vi "Nicolet 12 ICAI_gatefix3.vi"(3 "?":u16(ring)=10 items=["16", "32", "64", "128", "256", "512", "1024", "2048", "4096", "8192", "16384", "32768", "65536", "131072", "262144", "524288 (one channel)", ""], 5 "Sample Duration (sec)":u32(knob)=24 scale=1.0..33.0) -> (0 "Waveform Graph":waveform(dbl)[](graph)=[{"t0"=timestamp(0 s since 1904-01-01), "dt"=0.0001220703125, "Y"=array[40960 elements]}, {"t0"=timestamp(0 s since 1904-01-01), "dt"=0.0001220703125, "Y"=array[40960 elements]}], 2 "data":dbl[][](array[numeric]) format="%0.2f", 8 "points":i32=40960)   [LabVIEW 2010]
doc: "I. Description:\nThis example demonstrates how to acquire a finite amount of data (Waveform) using the DAQ device's internal clock, started by an analog edge condition.\n\nII. Instructions for Running:\n1. Select the physical channel to correspond to where your signal is input on the DAQ device.\n2. Enter the minimum and maximum voltage range.\nNote: For better accuracy try to match the input range to the expected voltage level of the measured signal.\n3. Set the number of samples to acquire per channel.\n4. Set the rate of the acquisition\nNote: The rate should be AT LEAST twice as fast as the maximum frequency component of the signal being acquired.\n5. Set the source of the start trigger. By default this is PFI0\n6. Set the slope and level of desired analog edge condition.\n\nIII. Block Diagram Steps:\n1. Create an empty task.\n2. Create an analog input voltage channel.\n3. Set the rate for the sample clock. Additionally, define the sample mode to be finite.\n4. Define the parameters for an Analog Slope Start Trigger.\n5. Call the Start VI to start the acquisition.\n6. Read all of the data.\n7. Stop the Analog Input Task.\n8. Call the Clear Task VI to clear the Task.\n9. Use the popup dialog box to display an error if any\nIV. I/O Connections Overview:\nMake sure your signal input terminal matches the Physical Channel I/O Control. In this case wire your signal to the ai0 pin on your DAQ Device."
uses:
  programs/Detection/200262.llb/Trigger Select.ctl
  <vilib>/Utility/error.llb/DialogType.ctl
  <vilib>/DAQmx/write.llb/DAQmx Write (Analog DBL 1Chan 1Samp).vi
  <vilib>/DAQmx/read.llb/DAQmx Read (Analog 2D DBL NChan NSamp).vi
  <vilib>/DAQmx/create/channels.llb/DAQmx Create Channel (AO-Voltage-Basic).vi
  <vilib>/daqmx/miscellaneous.llb/DAQmx Fill In Error Info.vi
  <vilib>/DAQmx/create/channels.llb/DAQmx Create Channel (AI-Voltage-Basic).vi
  <vilib>/DAQmx/configure/timing.llb/DAQmx Timing (Sample Clock).vi
  <vilib>/DAQmx/configure/trigger.llb/DAQmx Start Trigger (Analog Edge).vi
  <vilib>/DAQmx/configure/trigger.llb/DAQmx Reference Trigger (Digital Edge).vi
  <vilib>/measure/maspectr.llb/FFT Power Spectral Density for 1 Chan.vi
  <vilib>/measure/NI_MAPro.lvlib
  Program Files/National Instruments/LabVIEW 2010/resource/objmgr/daqmx.rc
panel:
  out "size(s)":i32[](array[numeric])
  in  "CAI/ICAI":bool=TRUE
  in  "?":path=path "C:/Users/Cardenas/Desktop/7_01/7_01_380fringe371mvmid_lockedat330.txt"
  in  "Path":path=path "C:/Users/Cardenas/Desktop/7_03/a6_200ms_span.txt"
  out "Time":dbl=5.5
  out "points pretriger":dbl=4096.0
  in  "Iterations to Average":i32=8
  in  "Sample Rate Hz":bool
  out "Cursor Time Selected":dbl=0.22413589186805782
  out "Cursor Peak to Peak Voltage":dbl=0.01024955436720143
  in  "Save Average To File":bool
  out "Pretrigger Samples":dbl=4096.0
  out "Seconds Per Division":dbl=0.1
  out "Posttrigger Samples Captured":dbl=40960.0
  in  "Voltage Offset":dbl(knob) scale=-2.0..2.0
  in  "Average / Live Display":bool
  in  "Seconds  Per Division":u32(knob) min=1 max=1 step=1 scale=0.0..15.0
  out "Samples Averaged":i32=3
  in  "?":bool=TRUE
  in  "Volts Per Division":dbl(knob)=0.5 scale=0.005..5.0
  in  "Pretrigger Duration (%)":dbl(knob)=0.1 min=0.0 max=2.0 step=1.0 scale=0.05..0.95
  in  "Analog Source":string="APFI0"
  in  "Digital External TTL Source":tag="/Dev1/PFI13"
  in  "Trigger Type":T1=enum."Digital Edge"
  in  "Analog Edge Level":dbl=-0.1 format="%0.2f"
  in  "Edge":i32(ring)=10280 items=["Rising"=10280, "Falling"=10171]
  in  "Physical Channel":tag="Dev1/ai22, Dev1/ai23" caption="Physical Channels"
  out "Sampling Iterations":i32=2
  in  "Maximum  Voltage":dbl=10.0
  in  "Minimum Voltage":dbl=-10.0
  out "Sampling Rate":i32=8192 caption="Sample Rate (Hz)"
  in  "stop":bool
  # "Channel\nConfiguration"
  # "Triggering Parameters"
  # "Voltage Parameters"
  # "TTL Trigger Options"
  # "Timing Parameters"
  # "External  Trigger Options"
  # "Storage Options"
  # "Nicolet 8.vi*If X scale markers are not drawn:\nRight click the waveform diagram -> select X axis -> marker spacing -> set to arbitrary AFTER\nsetting the correct seconds per division"
  # "CAI / ICAI"
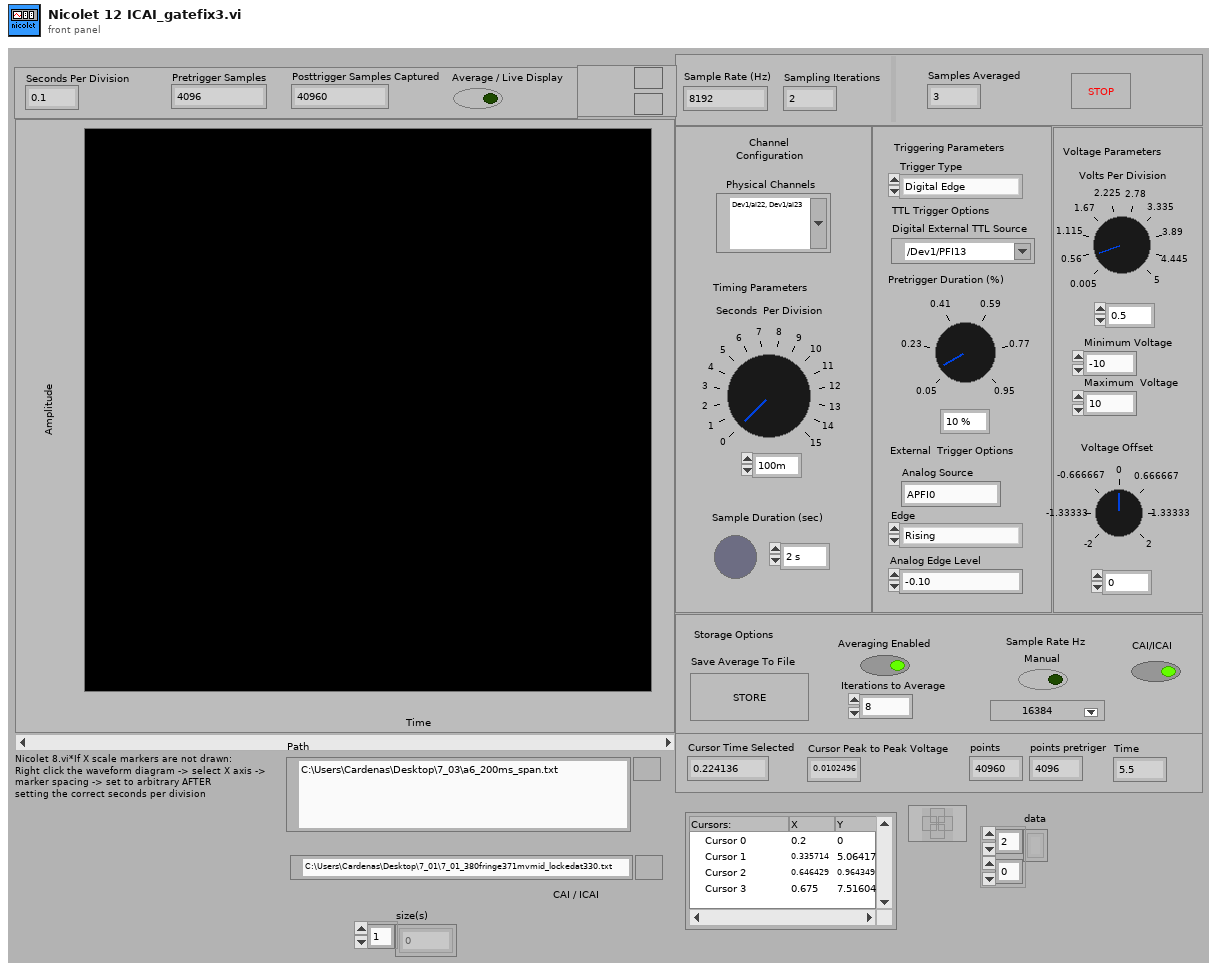
[diagram p1: front panel]
types:
  T1 = typedef "Trigger Select.ctl" = enum16{"None", "Analog Edge", "Digital Edge"}
  T2 = typedef "DialogType.ctl" = u16
  T3 = typedef "LVCursorListTypeDef.ctl" = cluster{"Name":string, "Color":u32, "Style":u8, "Point Style":u8, "Name Visible":bool, "Allow Drag":bool, "Cursor Mode":u32, "Plot":i32, "Index":i32, "Position":cluster{"X":dbl, "Y":dbl}, "X Scale":u32, "Y Scale":u32, "Watch Plots":i32[], "Watch All Plots":bool, "Plot Area":i32, "Label Offset":cluster{"X":dbl, "Y":dbl}}[]
  T4 = cluster{"Name":string, "Color":u32, "Style":u8, "Point Style":u8, "Name Visible":bool, "Allow Drag":bool, "Cursor Mode":u32, "Plot":i32, "Index":i32, "Position":cluster{"X":dbl, "Y":dbl}, "X Scale":u32, "Y Scale":u32, "Watch Plots":i32[], "Watch All Plots":bool, "Plot Area":i32, "Label Offset":cluster{"X":dbl, "Y":dbl}}
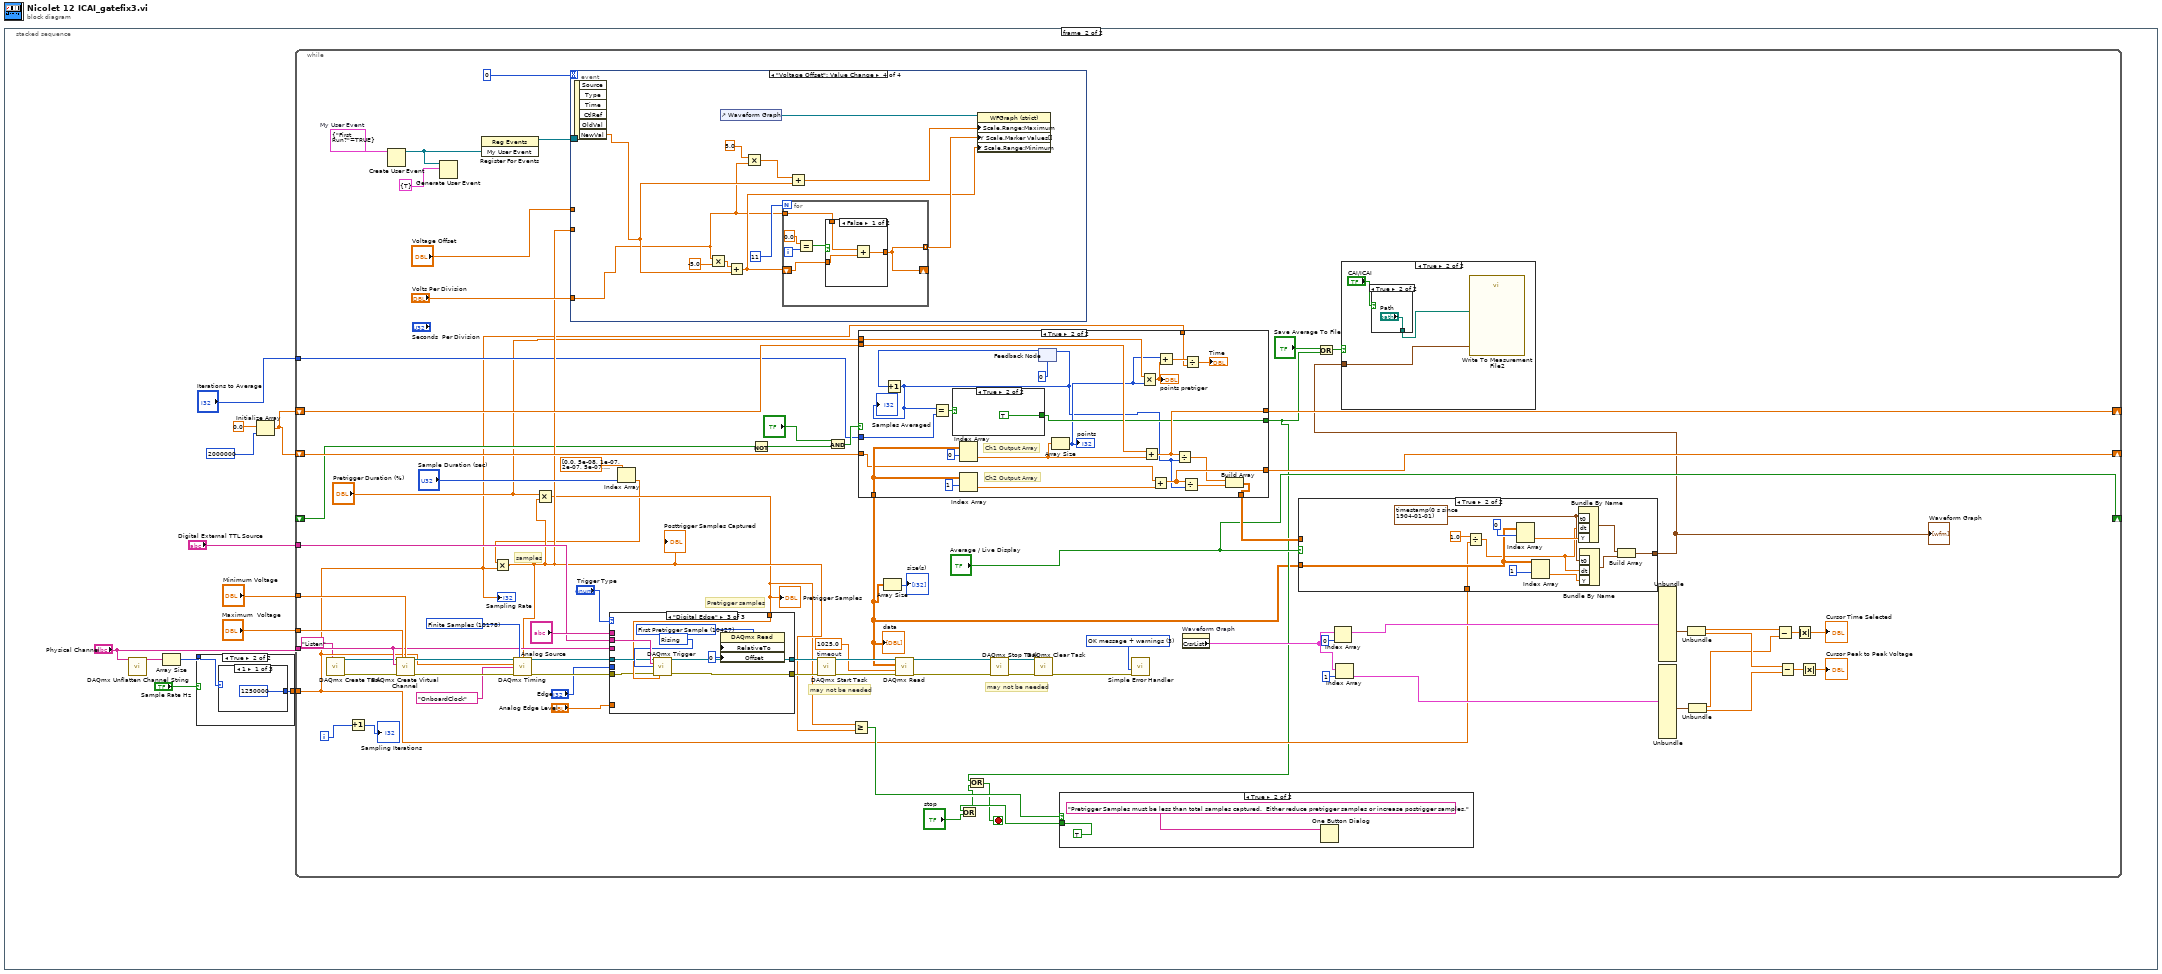
[diagram p0: block diagram]
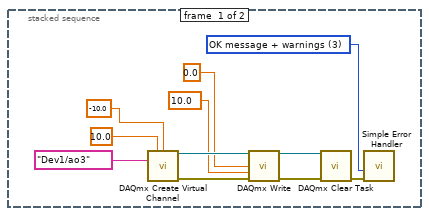
[diagram p2: hidden frame]
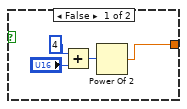
[diagram p3: hidden frame]
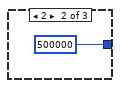
[diagram p4: hidden frame]
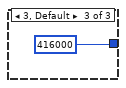
[diagram p5: hidden frame]
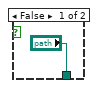
[diagram p7: hidden frame]
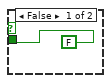
[diagram p8: hidden frame]
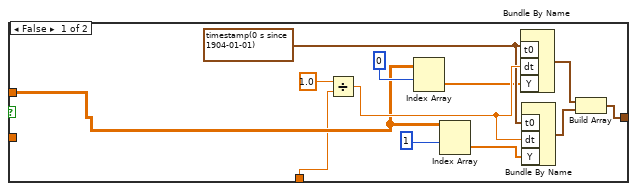
[diagram p9: hidden frame]
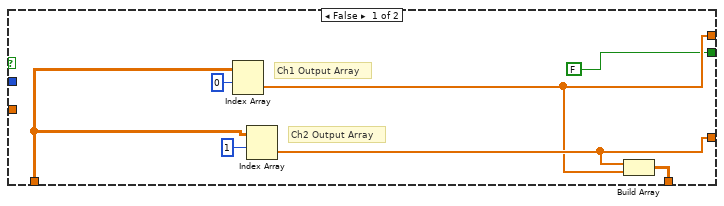
[diagram p10: hidden frame]
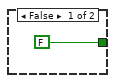
[diagram p11: hidden frame]
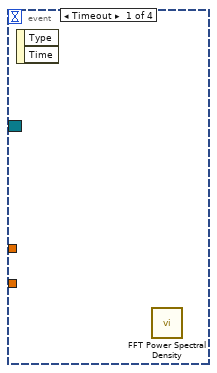
[diagram p12: hidden frame]
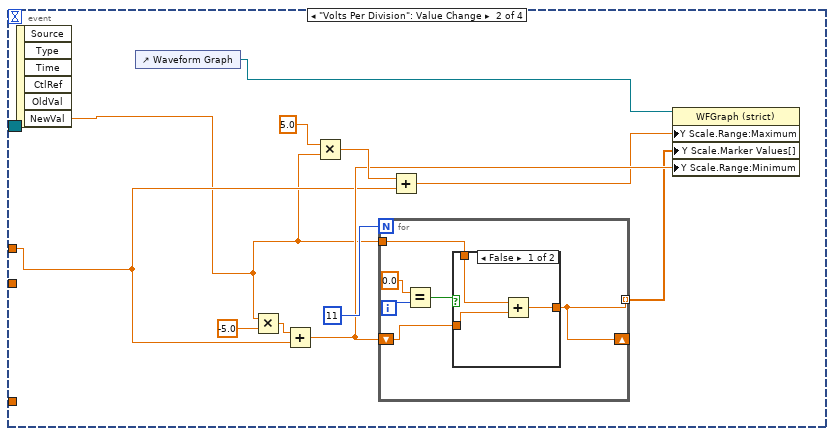
[diagram p13: hidden frame]
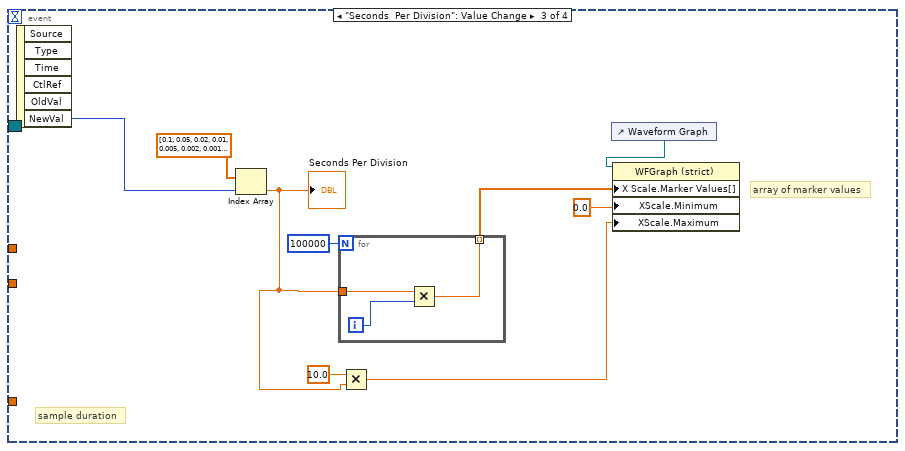
[diagram p15: hidden frame]
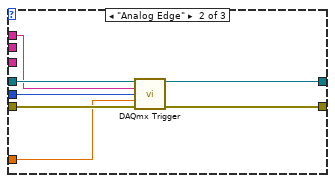
[diagram p18: hidden frame]
diagram:
  n1 = stacked-sequence {
    frame #0 {
      w4 = T2 3 items=["no dialog", "OK message", "continue or stop message", "OK message + warnings", "continue/stop + warnings"] ("type of dialog (OK msg:1)")
      n2 = call-poly <vilib>:"DAQmx Create Virtual Channel.vi"("maximum value"=10.0 ("Maximum Value"), "minimum value"=-10.0 ("Minimum Value"), "physical channels"=tag "Dev1/ao3" ("Physical Channel")) -> ("task out"=w7:refnum<k21>, "error out"=w8:errorcluster)  [unwired: 6 in, 5 out]
      n3 = call-poly <vilib>:"DAQmx Write.vi"("task/channels in"=w7, "data"=0.0 ("Voltage Output"), "timeout"=10.0, "error in"=w8) -> ("task out"=w2:refnum<k21>, "error out"=w3:errorcluster)  [unwired: 1 in, 9 out]
      n4 = call <vilib>:"DAQmx Clear Task.vi"("task in"=w2, "error in"=w3) -> ("error out"=w1:errorcluster)  [unwired: 13 out]
      n5 = call <vilib>:"Simple Error Handler.vi"("type of dialog (OK msg:1)"=w4, "error in (no error)"=w1) -> ()  [unwired: 8 out]
    }
    frame #1 {
      n6 = call <vilib>:"DAQmx Unflatten Channel String.vi"("names in"="Physical Channel") -> ("names out"=w19:string[])  [unwired: 1 in, 13 out]
      n7 = Array Size(array=w19) -> (size(s)=w17:i32)
      n8 = case shown="True" "Sample Rate Hz" {
        tunnel: [w25 w29] -> w18
        tunnel: w17 -> [_ w28]
        frame False {
          n9 = Add(x=4, y="?") -> (x+y=w26:i32)
          n10 = Power Of 2(x=w26) -> (2^x=w25:dbl)
        }
        frame True {
          n11 = case shown="1" w28 {
            tunnel: [1250000 500000 416000] -> w29
            frame 1 {
            }
            frame 2 {
            }
            frame 3, Default {
            }
          }
        }
      }
      n12 = Initialize Array(0.0, 2000000) -> (w12:dbl[])
      n13 = while {
        tunnel: "Minimum Voltage" -> [w94]
        tunnel: "Maximum  Voltage" -> [w93]
        tunnel: "Physical Channel" -> [w92]
        tunnel: "Digital External TTL Source" -> [w90]
        shift-right: [w84] -> _
        shift-left: w12 -> [w83]
        shift-right: [w79] -> _
        shift-left: w12 -> [w78]
        tunnel: w18 -> [w41]
        shift-right: ["Average / Live Display"] -> _
        shift-left: _ -> [w51]
        tunnel: "Iterations to Average" -> [w43]
        i -> [w37]
        stop <- w40 stop-if-true
        w89 = cluster{"First Run?":bool} {"First Run?"=TRUE}  # My User Event
        w109 = T2 3 items=["no dialog", "OK message", "continue or stop message", "OK message + warnings", "continue/stop + warnings"] ("type of dialog (OK msg:1)")
        w106 = 1025.0  # timeout
        w104 = 10178 items=["Finite Samples"=10178, "Continuous Samples"=10123] ("sample mode")
        # "samples"
        # "may not be needed"
        # "may not be needed"
        # "Pretrigger samples"
        n14 = call <vilib>:"DAQmx Create Task.vi"("new task name"="Listen") -> ("task out"=w82:refnum<k21>, "error out"=w81:errorcluster)  [unwired: 4 in, 9 out]
        n15 = Increment(x=w37) -> (x+1=→"Sampling Iterations":i32)
        n16 = Create User Event(user event datatype=w89) -> (user event=w87:refnum<user-event>)  [unwired: 1 in, 1 out]
        n17 = call-poly <vilib>:"DAQmx Create Virtual Channel.vi"("task in"=w82, "maximum value"=w93, "minimum value"=w94, "physical channels"=w92, "error in"=w81) -> ("task out"=w105:refnum<k21>, "error out"=w113:errorcluster)  [unwired: 4 in, 5 out]
        n18 = Generate User Event(user event=w87, event data cluster=cluster{"First Run?":bool} {"First Run?"=TRUE} ("event data")) -> ()  [unwired: 1 in, 2 out]
        n19 = register-events(w87) -> (reference out=w85:refnum<event-registration>)  [unwired: 2 in, 1 out]
        n20 = Index Array(array=dbl[] [0.0, 5e-08, 1e-07, 2e-07, 5e-07, 1e-06, 2e-06, 5e-06, 1e-05, 2e-05, 5e-05, 0.0001, 0.0002, 0.0005, 0.001, 0.002, 0.005, 0.01, 0.02, 0.05, 0.1, 0.2, 0.5, 1.0, 2.0, 5.0, 10.0, 16.5, 32.5, 65.0, 129.0, 257.0, 513.0, 1025.0], index="Sample Duration (sec)") -> (element=w48:dbl)
        n21 = Multiply(x=w48, y=w41) -> (x*y=w70:dbl)
        "Posttrigger Samples Captured" <- w70
        n22 = call-poly <vilib>:"DAQmx Timing.vi"("task/channels in"=w105, "sample mode"=w104, "samples per channel"=w70, "rate"=w41, "source"=tag "OnboardClock", "error in"=w113) -> ("task out"=w99:refnum<k21>, "error out"=w97:errorcluster)  [unwired: 1 in, 7 out]
        n23 = Multiply(x="Pretrigger Duration (%)", y=w70) -> (x*y=w69:dbl)
        "Pretrigger Samples" <- w69
        n24 = event shown="[3] \"Voltage Offset\": Value Change" {
          selector: w85 -> [_ _ _ _]
          dyn-events: _ -> [_ _ _ _]
          timeout: 0 -> [_ _ _ _]
          tunnel: w70 -> [_ _ _ _]
          tunnel: "Voltage Offset" -> [_ w181 _ _]
          tunnel: "Volts Per Division" -> [_ _ _ w213]
          event Timeout {
            n25 = event-data() -> ()  [unwired: 3 out]
            n26 = call-poly <vilib>:"FFT Power Spectral Density.vi"() -> ()  [unwired: 6 in, 6 out]
          }
          event "Volts Per Division": Value Change {
            n27 = event-data() -> ("NewVal"=w180:dbl)  [unwired: 6 out]
            n28 = control-ref of="Waveform Graph"() -> (w179:refnum<vi>)
            n29 = Multiply(x=w180, y=-5.0) -> (x*y=w186:dbl)
            n30 = Add(x=w186, y=w181) -> (x+y=w184:dbl)
            n31 = Multiply(x=5.0, y=w180) -> (x*y=w185:dbl)
            n32 = for {
              N: 11 -> [_]
              tunnel: w180 -> [w195]
              tunnel: [w194] -> w182 mode=indexing
              shift-right: [w194] -> _
              shift-left: w184 -> [w192]
              i -> [w190]
              n33 = Equal?(x=0.0, y=w190) -> (x = y?=w193:bool)
              n34 = case shown="False" w193 {
                tunnel: w195 -> [w198 _]
                tunnel: w192 -> [w197 w199]
                tunnel: [w196 w199] -> w194
                frame False {
                  n35 = Add(x=w198, y=w197) -> (x+y=w196:dbl)
                }
                frame True {
                }
              }
            }
            n36 = Add(x=w185, y=w181) -> (x+y=w183:dbl)
            n37 = property on="Property Node" class="WFGraph (strict)"(reference=w179, "Y Scale.Range:Maximum"=w183, "Y Scale.Marker Values[]"=w182, "Y Scale.Range:Minimum"=w184) -> ()  [unwired: 1 in, 2 out]
          }
          event "Seconds  Per Division": Value Change {
            # "sample duration"
            # "array of marker values"
            n38 = event-data() -> ("NewVal"=w207:u32)  [unwired: 6 out]
            n39 = Index Array(array=dbl[] [0.1, 0.05, 0.02, 0.01, 0.005, 0.002, 0.001, 0.0005, 0.0002, 0.0001, 5e-05, 2e-05, 1e-05, 5e-06, 2e-06, 1e-06], index=w207) -> (element=w201:dbl)
            "Seconds Per Division" <- w201
            n40 = for {
              N: 100000 -> [_]
              tunnel: w201 -> [w210]
              tunnel: [w209] -> w203 mode=indexing
              i -> [w211]
              n41 = Multiply(x=w210, y=w211) -> (x*y=w209:dbl)
            }
            n42 = Multiply(x=10.0, y=w201) -> (x*y=w200:dbl)
            n43 = control-ref of="Waveform Graph"() -> (w205:refnum<vi>)
            n44 = property on="Property Node" class="WFGraph (strict)"(reference=w205, "X Scale.Marker Values[]"=w203, "XScale.Minimum"=0.0 ("x"), "XScale.Maximum"=w200) -> ()  [unwired: 1 in, 2 out]
          }
          event "Voltage Offset": Value Change {
            n45 = event-data() -> ("NewVal"=w214:dbl)  [unwired: 6 out]
            n46 = Multiply(x=w213, y=-5.0) -> (x*y=w221:dbl)
            n47 = control-ref of="Waveform Graph"() -> (w212:refnum<vi>)
            n48 = Add(x=w221, y=w214) -> (x+y=w215:dbl)
            n49 = Multiply(x=5.0, y=w213) -> (x*y=w222:dbl)
            n50 = for {
              N: 11 -> [_]
              tunnel: w213 -> [w228]
              tunnel: [w227] -> w216 mode=indexing
              shift-right: [w227] -> _
              shift-left: w215 -> [w225]
              i -> [w223]
              n51 = Equal?(x=0.0, y=w223) -> (x = y?=w226:bool)
              n52 = case shown="False" w226 {
                tunnel: w228 -> [w231 _]
                tunnel: w225 -> [w230 w232]
                tunnel: [w229 w232] -> w227
                frame False {
                  n53 = Add(x=w231, y=w230) -> (x+y=w229:dbl)
                }
                frame True {
                }
              }
            }
            n54 = Add(x=w222, y=w214) -> (x+y=w217:dbl)
            n55 = property on="Property Node" class="WFGraph (strict)"(reference=w212, "Y Scale.Range:Maximum"=w217, "Y Scale.Marker Values[]"=w216, "Y Scale.Range:Minimum"=w215) -> ()  [unwired: 1 in, 2 out]
          }
        }
        n56 = case shown="\"Digital Edge\"" "Trigger Type" {
          tunnel: w99 -> [w234 w237 w248]
          tunnel: [w234 w239 w244] -> w98
          tunnel: w97 -> [w233 w241 w246]
          tunnel: [w233 w238 w251] -> w96
          tunnel: w92 -> [_ _ _]
          tunnel: "Analog Edge Level" -> [_ w240 _]
          tunnel: "Analog Source" -> [_ w236 _]
          tunnel: w90 -> [_ _ w250]
          tunnel: w69 -> [_ _ w247]
          tunnel: "Edge" -> [_ w235 _]
          frame "None", Default {
          }
          frame "Analog Edge" {
            n57 = call-poly <vilib>:"DAQmx Trigger.vi"("task/channels in"=w237, "source"=w236, "slope"=w235, "level"=w240, "error in"=w241) -> ("task out"=w239:refnum<k21>, "error out"=w238:errorcluster)  [unwired: 9 out]
          }
          frame "Digital Edge" {
            w242 = 10427 items=["First Sample"=10424, "Current Read Position"=10425, "Reference Trigger"=10426, "First Pretrigger Sample"=10427, "Most Recent Sample"=10428] ("RelativeTo")
            w249 = 10280 items=["Rising"=10280, "Falling"=10171] ("edge")
            n58 = call-poly <vilib>:"DAQmx Trigger.vi"("task/channels in"=w248, "source"=w250, "edge"=w249, "error in"=w246, "pretrigger samples per channel"=w247) -> ("task out"=w245:refnum<k21>, "error out"=w251:errorcluster)  [unwired: 9 out]
            n59 = property class="DAQmx Read"(reference=w245, "RelativeTo"=w242, "Offset"=0) -> (reference out=w244:refnum<k21>)  [unwired: 1 in, 1 out]
          }
        }
        n60 = Not(x=w51) -> (.not. x?=w50:bool)
        n61 = call <vilib>:"DAQmx Start Task.vi"("task/channels in"=w98, "error in"=w96) -> ("task out"=w107:refnum<k21>, "error out"=w112:errorcluster)  [unwired: 12 out]
        n62 = And(x="?", y=w50) -> (x .and. y?=w49:bool)
        n63 = Greater Or Equal?(x=w69, y=w70) -> (x >= y?=w73:bool)
        n64 = call-poly <vilib>:"DAQmx Read.vi"("task/channels in"=w107, "timeout"=w106, "error in"=w112) -> ("task out"=w103:refnum<k21>, "data"=w35:dbl[][], "error out"=w102:errorcluster)  [unwired: 1 in, 9 out]
        "data" <- w35
        n65 = case shown="True" w49 {
          tunnel: w35 -> [w150 w176]
          tunnel: [w148 w171] -> w84
          tunnel: w83 -> [_ w169]
          tunnel: [w149 w168] -> w79
          tunnel: w78 -> [_ w167]
          tunnel: [w147 w164] -> w68
          tunnel: [FALSE w162] -> w38
          tunnel: w43 -> [_ w160]
          tunnel: "Pretrigger Duration (%)" -> [_ w159]
          tunnel: w41 -> [_ w155]
          frame False {
            # "Ch2 Output Array"
            # "Ch1 Output Array"
            n66 = Index Array(array=w150, index (row)=0 ("disabled index (col)")) -> (element=w148:dbl[])  [unwired: 1 in]
            n67 = Index Array(array=w150, index (row)=1 ("disabled index (col)")) -> (element=w149:dbl[])  [unwired: 1 in]
            n68 = Build Array(w149, w148) -> (w147:dbl[][])
          }
          frame True {
            # "Ch2 Output Array"
            # "Ch1 Output Array"
            n69 = Index Array(array=w176, index (row)=0 ("disabled index (col)")) -> (element=w163:dbl[])  [unwired: 1 in]
            n70 = Index Array(array=w176, index (row)=1 ("disabled index (col)")) -> (element=w170:dbl[])  [unwired: 1 in]
            n71 = feedback #1(0) -> (w172:i32)
            n72 = Increment(x=w172) -> (x+1=w153:i32)
            "Samples Averaged" <- w153
            n73 = Equal?(x=w153, y=w160) -> (x = y?=w161:bool)
            n74 = case shown="True" w161 {
              tunnel: [FALSE TRUE] -> w162
              frame False {
              }
              frame True {
              }
            }
            n75 = feedback-in #1(w153) -> ()
            n76 = Array Size(array=w163) -> (size(s)=w158:i32)
            "points" <- w158
            n77 = Multiply(x=w159, y=w158) -> (x*y=w157:dbl)
            "points pretriger" <- w157
            n78 = Add(x=w169, y=w163) -> (x+y=w171:dbl[])
            n79 = Add(x=w167, y=w170) -> (x+y=w168:dbl[])
            n80 = Add(x=w158, y=w157) -> (x+y=w156:dbl)
            n81 = Divide(x=w171, y=w153) -> (x/y=w166:dbl[])
            n82 = Divide(x=w168, y=w153) -> (x/y=w165:dbl[])
            n83 = Divide(x=w156, y=w155) -> (x/y=→"Time":dbl)
            n84 = Build Array(w166, w165) -> (w164:dbl[][])
          }
        }
        n85 = Array Size(array=w35) -> (size(s)=→"size(s)":i32[])
        n86 = call <vilib>:"DAQmx Stop Task.vi"("task/channels in"=w103, "error in"=w102) -> ("task out"=w108:refnum<k21>, "error out"=w111:errorcluster)  [unwired: 12 out]
        n87 = call <vilib>:"DAQmx Clear Task.vi"("task in"=w108, "error in"=w111) -> ("error out"=w110:errorcluster)  [unwired: 13 out]
        n88 = case shown="True" w73 {
          tunnel: [FALSE TRUE] -> w71
          frame False {
          }
          frame True {
            n89 = One Button Dialog(message="Pretrigger Samples must be less than total samples captured.  Either reduce pretrigger samples or increase postrigger samples.") -> ()  [unwired: 2 out]
          }
        }
        n90 = Or(x=w71, y="stop") -> (x .or. y?=w39:bool)
        n91 = Or(x=w38, y=w39) -> (x .or. y?=w40:bool)
        n92 = call <vilib>:"Simple Error Handler.vi"("type of dialog (OK msg:1)"=w109, "error in (no error)"=w110) -> ()  [unwired: 8 out]
        n93 = property on="Waveform Graph" class="WFGraph (strict)"() -> ("CrsrList"=w47:T3)  [unwired: 2 in, 2 out]
        n94 = case shown="True" "Average / Live Display" {
          tunnel: w35 -> [_ w142]
          tunnel: [w124 w134] -> w46
          tunnel: w68 -> [w126 _]
          tunnel: w41 -> [w125 w138]
          frame False {
            w131 = timestamp(0 s since 1904-01-01) ("t0")
            n95 = Divide(x=1.0, y=w125) -> (x/y=w133:dbl)
            n96 = Index Array(array=w126, index (row)=0 ("disabled index (col)")) -> (element=w127:dbl[])  [unwired: 1 in]
            n97 = Index Array(array=w126, index (row)=1 ("disabled index (col)")) -> (element=w130:dbl[])  [unwired: 1 in]
            n98 = Bundle By Name("t0"=w131, "dt"=w133, "Y"=w127) -> (w122:waveform(dbl))  [unwired: 1 out]
            n99 = Bundle By Name("t0"=w131, "dt"=w133, "Y"=w130) -> (w123:waveform(dbl))  [unwired: 1 out]
            n100 = Build Array(w122, w123) -> (w124:waveform(dbl)[])
          }
          frame True {
            w140 = timestamp(0 s since 1904-01-01) ("t0")
            n101 = Divide(x=1.0, y=w138) -> (x/y=w137:dbl)
            n102 = Index Array(array=w142, index (row)=0 ("disabled index (col)")) -> (element=w145:dbl[])  [unwired: 1 in]
            n103 = Index Array(array=w142, index (row)=1 ("disabled index (col)")) -> (element=w141:dbl[])  [unwired: 1 in]
            n104 = Bundle By Name("t0"=w140, "dt"=w137, "Y"=w145) -> (w135:waveform(dbl))  [unwired: 1 out]
            n105 = Bundle By Name("t0"=w140, "dt"=w137, "Y"=w141) -> (w136:waveform(dbl))  [unwired: 1 out]
            n106 = Build Array(w135, w136) -> (w134:waveform(dbl)[])
          }
        }
        "Waveform Graph" <- w46
        n107 = Or(x="Save Average To File", y=w38) -> (x .or. y?=w45:bool)
        n108 = Index Array(array=w47, index=0) -> (element=w65:T4)
        n109 = Index Array(array=w47, index=1) -> (element=w64:T4)
        n110 = case shown="True" w45 {
          tunnel: w46 -> [_ w116]
          frame False {
          }
          frame True {
            n111 = case shown="True" "CAI/ICAI" {
              tunnel: ["?" "Path"] -> w115
              frame False {
              }
              frame True {
              }
            }
            n112 = call "Write To Measurement File2"("Signals"=w116, "Filename"=w115) -> ()  [unwired: 15 in, 3 out]
          }
        }
        n113 = Unbundle(w65) -> ("Position"=w63:cluster{"X":dbl, "Y":dbl})  [unwired: 15 out]
        n114 = Unbundle(w64) -> ("Position"=w62:cluster{"X":dbl, "Y":dbl})  [unwired: 15 out]
        n115 = Unbundle(w63) -> ("X"=w57:dbl, "Y"=w61:dbl)
        n116 = Unbundle(w62) -> ("X"=w55:dbl, "Y"=w60:dbl)
        n117 = Subtract(x=w57, y=w55) -> (x-y=w56:dbl)
        n118 = Subtract(x=w61, y=w60) -> (x-y=w59:dbl)
        n119 = Absolute Value(x=w56) -> (abs(x)=→"Cursor Time Selected":dbl)
        n120 = Absolute Value(x=w59) -> (abs(x)=→"Cursor Peak to Peak Voltage":dbl)
        "Sampling Rate" <- w41
      }
    }
  }
